vi "disconnect.vi"(4 "error in (no error)":errorcluster, 6 "Request data":variant, 7 "Python session in":refnum<k35>) -> (0 "error out":errorcluster, 2 "Response data":variant, 3 "Python session out":refnum<k35>)   [LabVIEW 2022 SP3]
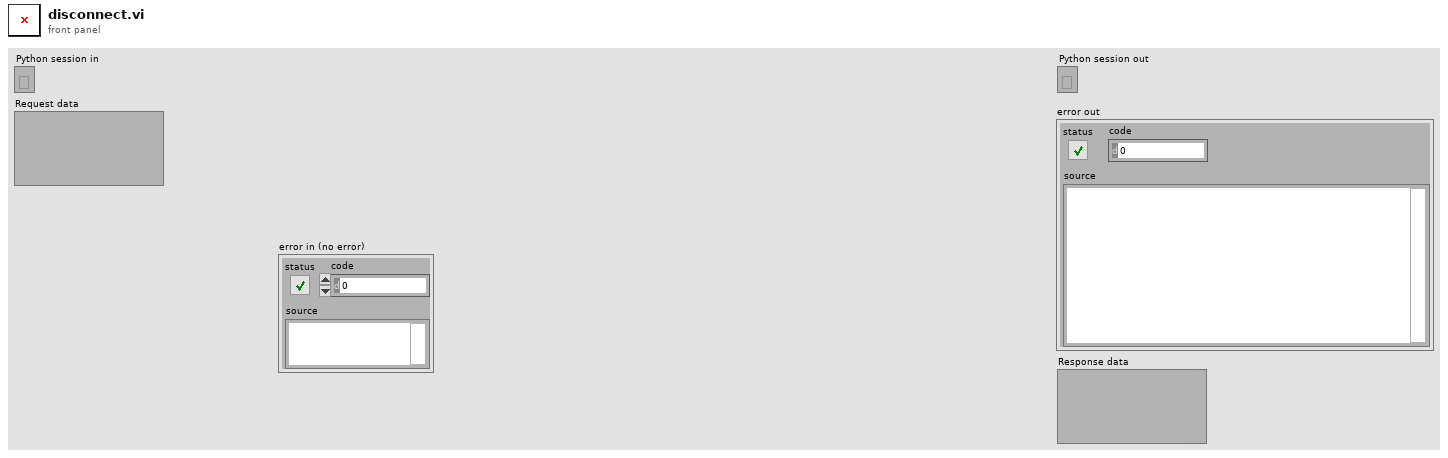
[diagram p1: front panel]
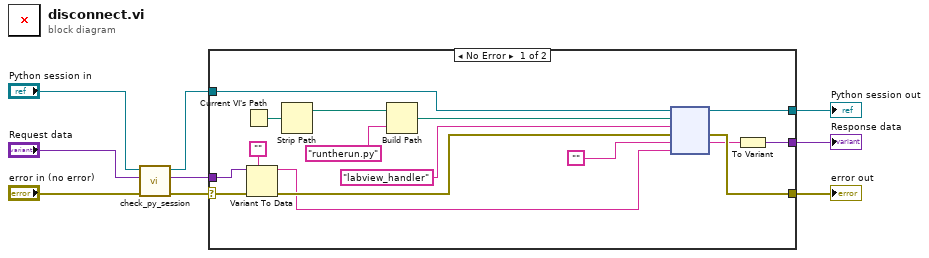
[diagram p0: block diagram]
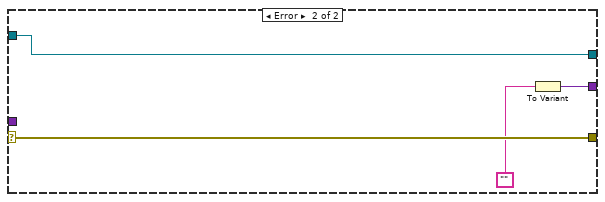
[diagram p2: hidden frame]
diagram:
  n1 = call "check_py_session.vi"("error in"="error in (no error)", "Request data"="Request data", "Python session in"="Python session in") -> ("error out"=w3:errorcluster, "Response data"=w4:variant, "Python session out"=w5:refnum<k35>)  [unwired: 2 in]
  n2 = case shown="No Error" w3 {
    selector: w3 -> [w15 w29]
    tunnel: w5 -> [w25 w28]
    tunnel: [w18 w28] -> w9
    tunnel: w4 -> [w16 _]
    tunnel: [w12 w29] -> w2
    tunnel: [w10 w26] -> w1
    frame No Error {
      n3 = Current VI's Path() -> (path=w20:path)
      n4 = Variant To Data(error in=w15, type="", Variant=w16) -> (data=w13:string, error out=w14:errorcluster)
      n5 = Strip Path(path=w20) -> (stripped path=w19:path)  [unwired: 1 out]
      n6 = Build Path(base path=w19, name or relative path="runtherun.py") -> (appended path=w22:path)
      n7 = node(w25, w22, "labview_handler" ("function name"), w14, "", w13) -> (w18:refnum<k35>, w12:errorcluster, w11:string)  [unwired: 1 in, 2 out]
      n8 = To Variant(anything=w11) -> (Variant=w10:variant)
    }
    frame Error {
      n9 = To Variant(anything="") -> (Variant=w26:variant)
    }
  }
  "error out" <- w2
  "Python session out" <- w9
  "Response data" <- w1
